vi "ConvertToLiA.vi"(8 "error in (no error)":errorcluster, 10 "Channel":u16(ring) items=["AO1"=1, "AO2"=2], 11 "Cluster":T3={"Start"=1.0, "Middle"=2.0, "End"=1.0, "Rate"=1.0, "Cycles"=0.0}) -> (0 "error out":errorcluster, 3 "Sweep":T1 {"Channel" items=["AO1"=1, "AO2"=2]; "Start" format="%#_6p"; "End" format="%#_6p"})   [LabVIEW 2020, in "MeasurementSMO.lvclass"]
uses:
  MeasurementSMO.lvclass
  <userlib>/LevyLab/Lockin-Multichannel/Lockin.DAQ/Typedefs/Sweep Pattern--Enum.ctl
  <userlib>/LevyLab/Lockin-Multichannel/Lockin.DAQ/Lockin.DAQ.lvclass
  <userlib>/LevyLab/Lockin-Multichannel/Instrument.Lockinl.UI/Typedefs/Sweep Channel--Cluster.ctl
  <userlib>/LevyLab/Lockin-Multichannel/Instrument.Lockinl.UI/Instrument.Lockin.UI.lvclass
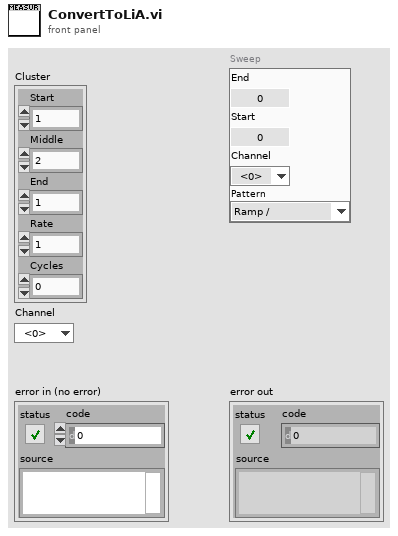
[diagram p1: front panel]
types:
  T1 = typedef "Instrument.Lockin.UI.lvclass/Sweep Channel--Cluster.ctl" = cluster{"End":dbl, "Start":dbl, "Channel":u16, "Pattern":T2}
  T2 = typedef "Lockin.DAQ.lvclass/Sweep Pattern--Enum.ctl" = enum16{"Ramp /", "Ramp /\\", "Smooth Ramp _/", "Smooth Ramp _/\\_", "Frequency"}
  T3 = cluster{"Start":dbl, "Middle":dbl, "End":dbl, "Rate":dbl, "Cycles":dbl}
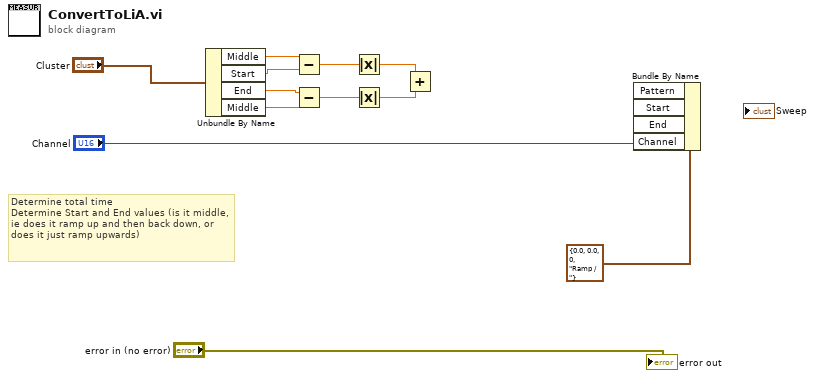
[diagram p0: block diagram]
diagram:
  # "Determine total time\nDetermine Start and End values (is it middle, ie does it ramp up and then back down, or does it just ramp upwards)"
  n1 = Unbundle By Name("Cluster") -> ("Middle"=w8:dbl, "Start"=w7:dbl, "End"=w6:dbl, "Middle"=w5:dbl)
  n2 = Subtract(x=w8, y=w7) -> (x-y=w4:dbl)
  n3 = Subtract(x=w6, y=w5) -> (x-y=w3:dbl)
  n4 = Absolute Value(x=w4) -> (abs(x)=w2:dbl)
  n5 = Absolute Value(x=w3) -> (abs(x)=w1:dbl)
  n6 = Add(x=w2, y=w1) -> ()  [unwired: 1 out]
  n7 = Bundle By Name(cluster=T1 {"End"=0.0, "Start"=0.0, "Channel"=0, "Pattern"=enum."Ramp /"} ("Sweep"), "Channel"="Channel") -> ()  [unwired: 3 in, 1 out]
  "error out" <- "error in (no error)"
